vi "UHR-Fleezers Control (host) - 10.8.vi"() -> ()   [LabVIEW 2014] (continued)
            n782 = property on="Trap 1 (ON/OFF)" class="Bool (strict)"("Val(Sgnl)"=w1188) -> ()  [unwired: 2 in, 2 out]
            n783 = property on="Trap 2 (ON/OFF)" class="Bool (strict)"("Val(Sgnl)"=w1188) -> ()  [unwired: 2 in, 2 out]
            n784 = call <vilib>:"Beep.vi"() -> ()  [unwired: 3 in, 9 out]
          }
          frame #5 {
            n785 = property on="Move Cap. 2 (ADig Top)" class="Bool (strict)"("Val(Sgnl)"=TRUE ("Value (Signaling)")) -> ()  [unwired: 2 in, 2 out]
            n786 = property on="Tab Control" class="TabCtl (strict)"("Val(Sgnl)"=T4."Status" ("Value (Signaling)")) -> ()  [unwired: 2 in, 2 out]
          }
        }
      }
      event "Dip for Protein": Value Change {
        n787 = event-data() -> ()  [unwired: 1 in, 5 out]
        n788 = case shown="True" "Dip for Protein" {
          tunnel: w1194 -> [_ w1196]
          tunnel: w1193 -> [_ w1195]
          frame False {
          }
          frame True {
            n789 = while {
              tunnel: w1196 -> [w1207]
              tunnel: w1195 -> [w1206]
              i -> [w1201]
              stop <- w1203 stop-if-true
              n790 = Increment(x=w1201) -> (x+1=→"Dip #":i32)
              n791 = flat-sequence {
                tunnel: w1206 -> [w1218]
                tunnel: w1207 -> [w1219]
                tunnel: [w1219] -> w1211
                tunnel: [w1218] -> w1210
                tunnel: [w1212] -> w1197
                tunnel: [w1224] -> w1205
                tunnel: [w1225] -> w1204
                tunnel: w1211 -> [w1226]
                tunnel: w1210 -> [w1227]
                tunnel: [w1222] -> w1198
                tunnel: w1197 -> [w1222]
                tunnel: [w1235] -> w1209
                tunnel: w1205 -> [w1235]
                tunnel: [w1234] -> w1208
                tunnel: w1204 -> [w1234]
                tunnel: [w1231] -> w1202
                tunnel: [w1230] -> w1199
                tunnel: w1198 -> [w1230]
                tunnel: w1208 -> [w1255]
                tunnel: w1209 -> [w1256]
                tunnel: w1202 -> [w1257]
                tunnel: w1199 -> [w1254]
                tunnel: [w1313] -> w1203
                frame #0 {
                  n792 = local read "Trap Pos. FB ON"() -> (w1212:bool)
                  n793 = Compound Arithmetic op=AND("Flow ON\nduring dip?", "FB OFF when \nflow ON", w1212) -> (w1213:bool)
                  n794 = case shown="True" "Move trap \nbefore dip move?" {
                    frame False {
                    }
                    frame True {
                      n795 = property on="Trap Delta (MHz)" class="DigNum (strict)"("Val(Sgnl)"="Dipping Delta (MHz)") -> ()  [unwired: 2 in, 2 out]
                    }
                  }
                  n796 = property on="Green Laser ON/Interlacing" class="Bool (strict)"("Val(Sgnl)"="Green ON\nbefore dip?") -> ()  [unwired: 2 in, 2 out]
                  n797 = property on="Sample Channel\nFlow" class="Bool (strict)"("Val(Sgnl)"="Flow ON\nduring dip?") -> ()  [unwired: 2 in, 2 out]
                  n798 = case shown="True" w1213 {
                    frame False {
                    }
                    frame True {
                      n799 = property on="Trap Pos. FB ON" class="Bool (strict)"("Val(Sgnl)"=FALSE ("Value (Signaling)")) -> ()  [unwired: 2 in, 2 out]
                    }
                  }
                }
                frame #1 {
                  n800 = local read "Saved Stage Positions"() -> (w1229:dbl[][])
                  n801 = local write "Cancel dwell"(FALSE ("Cancel dwell")) -> ()
                  n802 = call "move to saved stage position.vi"("error in"=w1227, "Stage VISA resource name in"=w1226, "Position"="Dip Stage \nPosition", "Saved Stage Positions"=w1229) -> ("VISA resource name out"=w1224:refnum<visa-resource-name>, "error out"=w1225:errorcluster)
                }
                frame #2 {
                  n803 = node-c288() -> (w1233:T21)  [unwired: 4 in]
                  n804 = timed-loop {
                    timing: w1233 -> [_]
                    timing-out: [_] -> w1232
                    tunnel: [w1239] -> w1231
                    i -> [w1236]
                    stop <- w1240 stop-if-true
                    n805 = node-c288() -> ()  [unwired: 1 in, 1 out]
                    n806 = Greater Or Equal?(x=w1236, y="Dip Duration (s)") -> (x >= y?=w1248:bool)
                    n807 = local read "Dip for Protein"() -> (w1241:bool)
                    n808 = local read "Dump Beads"() -> (w1238:bool)
                    n809 = local read "Cancel dwell"() -> (w1247:bool)
                    n810 = local read "Pause dwell"() -> (w1244:bool)
                    n811 = Not(x=w1241) -> (.not. x?=w1246:bool)
                    n812 = Compound Arithmetic op=OR(w1247, w1248, w1246) -> (w1245:bool)
                    n813 = Select(t=FALSE, s=w1244, f=w1245) -> (s? t:f=w1242:bool)
                    n814 = Not(x=w1238) -> (.not. x?=w1237:bool)
                    n815 = node-c288() -> ()  [unwired: 1 in, 1 out]
                    n816 = And(x=w1241, y=w1237) -> (x .and. y?=w1239:bool)
                    n817 = Or(x=w1242, y=w1238) -> (x .or. y?=w1240:bool)
                    "Dip Time (s)" <- w1236
                  }
                  n818 = node-c288(w1232) -> ()  [unwired: 1 out]
                }
                frame #3 {
                  n819 = case shown="True" w1257 {
                    tunnel: w1256 -> [_ w1262]
                    tunnel: w1255 -> [_ w1261]
                    tunnel: w1254 -> [_ w1258]
                    frame False {
                    }
                    frame True {
                      n820 = flat-sequence {
                        tunnel: w1261 -> [w1266]
                        tunnel: w1262 -> [w1267]
                        tunnel: [w1267] -> w1260
                        tunnel: [w1266] -> w1259
                        tunnel: w1258 -> [w1263]
                        tunnel: w1260 -> [w1277]
                        tunnel: w1259 -> [w1276]
                        tunnel: w1258 -> [w1285]
                        frame #0 {
                          n821 = local read "Sample Channel\nFlow"() -> (w1265:bool)
                          n822 = case shown="False" w1265 {
                            tunnel: "Flow ON \nduring return\nfrom dip?" -> [w1268 w1271]
                            tunnel: w1263 -> [_ w1270]
                            frame False {
                              n823 = case shown="True" w1268 {
                                frame False {
                                }
                                frame True {
                                n824 = property on="Sample Channel\nFlow" class="Bool (strict)"("Val(Sgnl)"=TRUE ("Value (Signaling)")) -> ()  [unwired: 2 in, 2 out]
                                }
                              }
                            }
                            frame True {
                              n825 = case shown="False" w1271 {
                                tunnel: w1270 -> [w1272 _]
                                frame False {
                                n826 = property on="Trap Pos. FB ON" class="Bool (strict)"("Val(Sgnl)"=w1272) -> ()  [unwired: 2 in, 2 out]
                                n827 = property on="Sample Channel\nFlow" class="Bool (strict)"("Val(Sgnl)"=FALSE ("Value (Signaling)")) -> ()  [unwired: 2 in, 2 out]
                                }
                                frame True {
                                }
                              }
                            }
                          }
                        }
                        frame #1 {
                          # "For turning on green laser before stage reaches lower spot"
                          n828 = case shown="True" "Green ON\nafter start\nreturn?" {
                            frame False {
                            }
                            frame True {
                              n829 = flat-sequence {
                                frame #0 {
                                n830 = Multiply(x="Green delay after \nstart return (s)", y=1000.0) -> (x*y=w1282:dbl)
                                n831 = Wait (ms)(milliseconds to wait=w1282) -> ()  [unwired: 1 out]
                                }
                                frame #1 {
                                n832 = property on="Green Laser ON/Interlacing" class="Bool (strict)"("Val(Sgnl)"=TRUE ("Value (Signaling)")) -> ()  [unwired: 2 in, 2 out]
                                }
                              }
                            }
                          }
                          n833 = local read "Saved Stage Positions"() -> (w1280:dbl[][])
                          n834 = local write "Cancel dwell"(FALSE ("Cancel dwell")) -> ()
                          n835 = call "move to saved stage position.vi"("error in"=w1276, "Stage VISA resource name in"=w1277, "Position"="Return Stage \nPosition", "Saved Stage Positions"=w1280) -> ("error out"=w1278:errorcluster)  [unwired: 1 out]
                          n836 = local write "Stage Control Serial Error"(w1278) -> ()
                        }
                        frame #2 {
                          n837 = property on="Trap Pos. FB ON" class="Bool (strict)"("Val(Sgnl)"=w1285) -> ()  [unwired: 2 in, 2 out]
                          n838 = case shown="True" "Green ON \nafter return?" {
                            frame False {
                            }
                            frame True {
                              n839 = property on="Green Laser ON/Interlacing" class="Bool (strict)"("Val(Sgnl)"=TRUE ("Value (Signaling)")) -> ()  [unwired: 2 in, 2 out]
                            }
                          }
                          n840 = case shown="True" "Move trap after return?" {
                            frame False {
                            }
                            frame True {
                              n841 = property on="Trap Delta (MHz)" class="DigNum (strict)"("Val(Sgnl)"="Dip Trap Delta 2 (MHz)") -> ()  [unwired: 2 in, 2 out]
                            }
                          }
                          n842 = case shown="True" "Save data after return?" {
                            frame False {
                            }
                            frame True {
                              n843 = property on="Start Saving" class="Bool (strict)"("Val(Sgnl)"=TRUE ("Value (Signaling)")) -> ()  [unwired: 2 in, 2 out]
                            }
                          }
                          n844 = property on="Sample Channel\nFlow" class="Bool (strict)"("Val(Sgnl)"="Flow ON\nduring daq?") -> ()  [unwired: 2 in, 2 out]
                        }
                        frame #3 {
                          n845 = node-c288() -> (w1294:T21)  [unwired: 4 in]
                          n846 = timed-loop {
                            timing: w1294 -> [_]
                            timing-out: [_] -> w1293
                            i -> [w1295]
                            stop <- w1297 stop-if-true
                            n847 = node-c288() -> ()  [unwired: 1 in, 1 out]
                            n848 = local read "Dump Beads"() -> (w1296:bool)
                            n849 = Greater Or Equal?(x=w1295, y="Dwell Duration (s)") -> (x >= y?=w1302:bool)
                            n850 = local read "Dip for Protein"() -> (w1299:bool)
                            n851 = Not(x=w1299) -> (.not. x?=w1298:bool)
                            n852 = Compound Arithmetic op=OR(w1302, "Cancel dwell", w1298) -> (w1301:bool)
                            n853 = node-c288() -> ()  [unwired: 1 in, 1 out]
                            n854 = Select(t=FALSE, s="Pause dwell", f=w1301) -> (s? t:f=w1304:bool)
                            n855 = Or(x=w1304, y=w1296) -> (x .or. y?=w1297:bool)
                            "Dwell Time (s)" <- w1295
                          }
                          n856 = node-c288(w1293) -> ()  [unwired: 1 out]
                        }
                      }
                    }
                  }
                }
                frame #4 {
                  n857 = local read "Dip for Protein"() -> (w1314:bool)
                  n858 = local read "Dump Beads"() -> (w1311:bool)
                  n859 = local write "Cancel dwell"(FALSE ("Cancel dwell")) -> ()
                  n860 = Not(x=w1314) -> (.not. x?=w1315:bool)
                  n861 = Not(x="Cont. Repeat Dipping?") -> (.not. x?=w1317:bool)
                  n862 = Compound Arithmetic op=OR(w1315, w1317, w1311) -> (w1313:bool)
                }
              }
            }
          }
        }
      }
      event "Profile": Value Change {
        n863 = event-data() -> ()  [unwired: 1 in, 5 out]
        n864 = flat-sequence {
          tunnel: w1326 -> [w1329]
          tunnel: w1325 -> [w1337]
          tunnel: [w1331] -> w1324
          tunnel: [w1330] -> w1323
          tunnel: [w1328] -> w1321
          tunnel: [w1327] -> w1318
          tunnel: w1324 -> [w1344]
          tunnel: w1323 -> [w1343]
          tunnel: [w1341] -> w1322
          tunnel: w1321 -> [w1342]
          tunnel: [w1340] -> w1320
          tunnel: [w1339] -> w1319
          tunnel: w1318 -> [w1339]
          tunnel: w1322 -> [w1348]
          tunnel: w1320 -> [w1347]
          tunnel: w1319 -> [w1346]
          frame #0 {
            n865 = call "Read Stage Position.vi"("error in"=w1337, "VISA resource name in"=w1329) -> ("Current Position"=w1327:cluster{dbl, dbl, dbl}, "error out"=w1330:errorcluster, "VISA resource name out"=w1328:refnum<visa-resource-name>)  [unwired: 1 out]
            "Current Position" <- w1327
            n866 = local write "Stage Control Serial Error"(w1330) -> ()
            n867 = Unbundle(w1327) -> (w1334:dbl, w1336:dbl, w1332:dbl)
            n868 = Add(x=w1336, y="Y change (mm)") -> (x+y=w1333:dbl)
            n869 = Bundle(w1334, w1333, w1332) -> (w1331:cluster{dbl, dbl, dbl})  [unwired: 1 in]
          }
          frame #1 {
            # "move to new position and start saving"
            n870 = local write "Stage Moving"(TRUE ("Stage Moving")) -> ()
            n871 = local write "Start Saving"(TRUE ("Start Saving")) -> ()
            n872 = call "Set Stage Position.vi"("Position"=w1344, "error in"=w1343, "VISA resource name in"=w1342) -> ("error out"=w1340:errorcluster, "VISA resource name out"=w1341:refnum<visa-resource-name>)  [unwired: 1 out]
          }
          frame #2 {
            # "go back to start"
            n873 = call "Set Stage Position.vi"("Position"=w1346, "error in"=w1347, "VISA resource name in"=w1348) -> ()  [unwired: 3 out]
          }
          frame #3 {
            # "stop saving"
            n874 = local write "Stop Saving"(TRUE ("Stop Saving")) -> ()
            n875 = local write "Stage Moving"(FALSE ("Stage Moving")) -> ()
          }
        }
      }
      event "Move to Position 1", "Move to Position 2", "Move to Position 3", "Move to Position 4", "Move to Position 5", "Lower Ch. Cap.": Value Change {
        n876 = event-data() -> ()  [unwired: 1 in, 5 out]
        n877 = Or(x="Move to Position 5", y="Lower Ch. Cap.") -> (x .or. y?=w1354:bool)
        n878 = Build Array("Move to Position 1", "Move to Position 2", "Move to Position 3", "Move to Position 4", w1354) -> (w1357:bool[])
        n879 = Boolean Array To Number(Boolean array=w1357) -> (number=w1356:u32)
        n880 = Logarithm Base 2(1:w1356) -> (0:w1355:dbl)
        n881 = flat-sequence {
          tunnel: w1355 -> [w1366]
          tunnel: w1352 -> [w1364]
          tunnel: w1351 -> [w1363]
          frame #0 {
            n882 = local read "Saved Stage Positions"() -> (w1374:dbl[][])
            n883 = Array Subset(array=w1374, index (row)=w1366, length (row)=1 ("length"), index (col)=1 ("index"), length (col)=3 ("length")) -> (w1371:dbl[][])
            n884 = Reshape Array(w1371, 3 ("dimension size")) -> (w1369:dbl[])
            n885 = Array To Cluster(array=w1369) -> (cluster=w1368:cluster{"[0]":dbl, "[1]":dbl, "[2]":dbl})
            n886 = call "Set Stage Position.vi"("Position"=w1368, "error in"=w1363, "VISA resource name in"=w1364) -> ("error out"=w1367:errorcluster)  [unwired: 2 out]
            n887 = local write "Stage Moving"(TRUE ("Stage Moving")) -> ()
            n888 = local write "Stage Control Serial Error"(w1367) -> ()
          }
          frame #1 {
            n889 = local write "Stage Moving"(FALSE ("Stage Moving")) -> ()
            n890 = call <vilib>:"Beep.vi"() -> ()  [unwired: 3 in, 9 out]
          }
        }
      }
      event "Got ADig bead": Value Change {
        n891 = event-data() -> ()  [unwired: 1 in, 5 out]
        n892 = flat-sequence {
          frame #0 {
            n893 = local read "Cap 1 Samp Flow ON"() -> (w1378:bool)
            n894 = case shown="True" w1378 {
              frame False {
              }
              frame True {
                n895 = property on="Sample Channel\nFlow" class="Bool (strict)"("Val(Sgnl)"=TRUE ("Value (Signaling)")) -> ()  [unwired: 2 in, 2 out]
              }
            }
          }
          frame #1 {
            n896 = property on="Inject Pump 3" class="Bool (strict)"("Val(Sgnl)"=FALSE ("Value (Signaling)")) -> ()  [unwired: 2 in, 2 out]
          }
          frame #2 {
            n897 = property on="Move Cap. 1 (DNA Bottom)" class="Bool (strict)"("Val(Sgnl)"=TRUE ("Value (Signaling)")) -> ()  [unwired: 2 in, 2 out]
          }
        }
      }
      event "Force FB Data\nScript": Value Change {
        n898 = event-data() -> ()  [unwired: 1 in, 5 out]
        n899 = flat-sequence {
          tunnel: w1387 -> [w1391]
          tunnel: w1388 -> [w1392]
          tunnel: [w1392] -> w1383
          tunnel: [w1391] -> w1382
          tunnel: w1383 -> [w1395]
          tunnel: w1382 -> [w1394]
          tunnel: ["Trap Trig Fl."] -> w1384
          tunnel: [w1420] -> w1385
          tunnel: w1384 -> [w1420]
          tunnel: [w1424] -> w1386
          tunnel: w1385 -> [w1424]
          tunnel: w1386 -> [w1426]
          frame #0 {
            n900 = property on="Trap Delta (MHz)" class="DigNum (strict)"("Val(Sgnl)"="Trap Delta Before Moving") -> ()  [unwired: 2 in, 2 out]
          }
          frame #1 {
            n901 = local read "Saved Stage Positions"() -> (w1397:dbl[][])
            n902 = local write "FB Trap Pos Offset"(0.0 ("FB Trap Pos Offset")) -> ()
            n903 = property on="Trap Pos. FB Offset Factor" class="DigNum (strict)"("Val(Sgnl)"=i64 0 ("Value (Signaling)")) -> ()  [unwired: 2 in, 2 out]
            n904 = local write "Stage Moving"(TRUE ("Stage Moving")) -> ()
            n905 = call "move to saved stage position.vi"("error in"=w1394, "Stage VISA resource name in"=w1395, "Position"="Stage Position To Establish FB", "Saved Stage Positions"=w1397) -> ("error out"=w1393:errorcluster)  [unwired: 1 out]
            n906 = local write "Stage Control Serial Error"(w1393) -> ()
          }
          frame #2 {
            n907 = call <vilib>:"Beep.vi"() -> ()  [unwired: 3 in, 9 out]
            n908 = Multiply(x="Wait (s)", y=u32 1000 ("milliseconds to wait")) -> (x*y=w1403:u32)
            n909 = property on="Trap Delta (MHz)" class="DigNum (strict)"("Val(Sgnl)"="Starting \nTrap Delta (MHz)") -> ()  [unwired: 2 in, 2 out]
            n910 = local write "Stage Moving"(FALSE ("Stage Moving")) -> ()
            n911 = Wait (ms)(milliseconds to wait=w1403) -> ()  [unwired: 1 out]
            n912 = property on="Tab Control 2" class="TabCtl (strict)"("Val(Sgnl)"=T6."Feedback on Trap Position" ("Value (Signaling)")) -> ()  [unwired: 2 in, 2 out]
            n913 = property on="Tab Control" class="TabCtl (strict)"("Val(Sgnl)"=T4."Trap Control (RF)" ("Value (Signaling)")) -> ()  [unwired: 2 in, 2 out]
          }
          frame #3 {
            n914 = property on="Set Reading to\nSetpoint" class="Bool (strict)"("Val(Sgnl)"=TRUE ("Value (Signaling)")) -> ()  [unwired: 2 in, 2 out]
            n915 = Wait (ms)(milliseconds to wait=u32 500) -> ()  [unwired: 1 out]
          }
          frame #4 {
            n916 = property on="Trap Pos. FB ON" class="Bool (strict)"("Val(Sgnl)"=TRUE ("Value (Signaling)")) -> ()  [unwired: 2 in, 2 out]
            n917 = Wait (ms)(milliseconds to wait=u32 250) -> ()  [unwired: 1 out]
          }
          frame #5 {
            n918 = case shown="False" "Trap Trig Fl." {
              frame False {
                n919 = case shown="True" "Green ON after FB ON?" {
                  selector: "Green ON after FB ON?" -> [_ w1419]
                  frame False {
                  }
                  frame True {
                    n920 = property on="Green Laser ON/Interlacing" class="Bool (strict)"("Val(Sgnl)"=w1419) -> ()  [unwired: 2 in, 2 out]
                  }
                }
              }
              frame True {
              }
            }
            n921 = case shown="True" "Remove Action Offset" {
              tunnel: TRUE ("Value (Signaling)") -> [w1416 w1417]
              frame False {
                n922 = property on="Remove Unwinding Offset" class="Bool (strict)"("Val(Sgnl)"=w1416) -> ()  [unwired: 2 in, 2 out]
              }
              frame True {
                n923 = property on="Remove Action Offset" class="Bool (strict)"("Val(Sgnl)"=w1417) -> ()  [unwired: 2 in, 2 out]
              }
            }
            n924 = Wait (ms)(milliseconds to wait=u32 250) -> ()  [unwired: 1 out]
          }
          frame #6 {
            n925 = property on="Start Saving" class="Bool (strict)"("Val(Sgnl)"=TRUE ("Value (Signaling)")) -> ()  [unwired: 2 in, 2 out]
            n926 = Wait (ms)(milliseconds to wait=u32 5000) -> ()  [unwired: 1 out]
          }
          frame #7 {
            w1423 = TRUE ("Value (Signaling)")
            n927 = property on="Rem fb disp offset" class="Bool (strict)"("Val(Sgnl)"=w1423) -> ()  [unwired: 2 in, 2 out]
            n928 = property on="Remove Offset" class="Bool (strict)"("Val(Sgnl)"=w1423) -> ()  [unwired: 2 in, 2 out]
            n929 = Wait (ms)(milliseconds to wait=u32 100) -> ()  [unwired: 1 out]
          }
          frame #8 {
            n930 = case shown="True" w1426 {
              frame False {
              }
              frame True {
                n931 = local write "Trap Trig. Fl."(TRUE ("Value (Signaling)")) -> ()
              }
            }
          }
          frame #9 {
            n932 = case shown="True" "Start dipping after?" {
              frame False {
              }
              frame True {
                n933 = flat-sequence {
                  frame #0 {
                    n934 = Multiply(x="Delay before dipping (s)", y=1000.0) -> (x*y=w1430:dbl)
                    n935 = Wait (ms)(milliseconds to wait=w1430) -> ()  [unwired: 1 out]
                  }
                  frame #1 {
                    n936 = property on="Dip for Protein" class="Bool (strict)"("Val(Sgnl)"=TRUE ("Value (Signaling)")) -> ()  [unwired: 2 in, 2 out]
                    n937 = local write "Scripts"(T1."Dipping" ("Scripts")) -> ()
                  }
                }
              }
            }
          }
        }
      }
      event "Fixed Traps Data\nScript": Value Change {
        n938 = event-data() -> ()  [unwired: 1 in, 5 out]
        n939 = flat-sequence {
          frame #0 {
            n940 = case shown="True" "Green ON" {
              frame False {
              }
              frame True {
                n941 = property on="Green Laser ON/Interlacing" class="Bool (strict)"("Val(Sgnl)"=TRUE) -> ()  [unwired: 2 in, 2 out]
              }
            }
            n942 = local write "Offset (nm)"(0.0 ("Offset (nm)")) -> ()
            n943 = property on="Sample Channel\nFlow" class="Bool (strict)"("Val(Sgnl)"=FALSE ("Value (Signaling)")) -> ()  [unwired: 2 in, 2 out]
            n944 = property on="Trap Delta (MHz)" class="DigNum (strict)"("Val(Sgnl)"="Fixed Traps Trap Delta (MHz)") -> ()  [unwired: 2 in, 2 out]
          }
          frame #1 {
            n945 = Wait (ms)(milliseconds to wait=u32 1000) -> ()  [unwired: 1 out]
          }
          frame #2 {
            n946 = local write "Start Saving"(TRUE ("Start Saving")) -> ()
          }
          frame #3 {
            n947 = local read "Bead Sep. Int. Time (s)"() -> (w1441:dbl)
            n948 = Multiply(x=w1441, y=1000.0) -> (x*y=w1443:dbl)
            n949 = Wait (ms)(milliseconds to wait=w1443) -> ()  [unwired: 1 out]
          }
          frame #4 {
            n950 = property on="Remove Offset" class="Bool (strict)"("Val(Sgnl)"=TRUE ("Value (Signaling)")) -> ()  [unwired: 2 in, 2 out]
          }
          frame #5 {
            n951 = property on="Dip for Protein" class="Bool (strict)"("Val(Sgnl)"="Start dipping after?") -> ()  [unwired: 2 in, 2 out]
          }
        }
      }
      event "Got DNA bead": Value Change {
        n952 = event-data() -> ()  [unwired: 1 in, 5 out]
        n953 = flat-sequence {
          frame #0 {
            n954 = local read "Daq spot flow on"() -> (w1448:bool)
            n955 = case shown="True" w1448 {
              frame False {
              }
              frame True {
                n956 = property on="Sample Channel\nFlow" class="Bool (strict)"("Val(Sgnl)"=TRUE ("Value (Signaling)")) -> ()  [unwired: 2 in, 2 out]
              }
            }
            n957 = property on="Got DNA bead" class="Bool"("Key Focus"=FALSE) -> ()  [unwired: 2 in, 2 out]
          }
          frame #1 {
            n958 = property on="Inject Pump 1" class="Bool (strict)"("Val(Sgnl)"=FALSE ("Value (Signaling)")) -> ()  [unwired: 2 in, 2 out]
          }
          frame #2 {
            n959 = property on="Cal/Data Acq. Spot" class="Bool (strict)"("Val(Sgnl)"=TRUE ("Value (Signaling)")) -> ()  [unwired: 2 in, 2 out]
          }
        }
      }
      event "Take Stepping Data": Value Change {
        n960 = event-data() -> ()  [unwired: 1 in, 5 out]
        n961 = local read "Save ave N"() -> (w1460:dbl)
        n962 = flat-sequence {
          tunnel: w1460 -> [w1462]
          tunnel: [w1462] -> w1455
          tunnel: [w1464] -> w1456
          tunnel: w1455 -> [w1464]
          tunnel: [w1466] -> w1457
          tunnel: w1456 -> [w1466]
          tunnel: [w1469] -> w1458
          tunnel: w1457 -> [w1469]
          tunnel: [w1471] -> w1459
          tunnel: w1458 -> [w1471]
          tunnel: [w1473] -> w1453
          tunnel: w1459 -> [w1473]
          tunnel: w1453 -> [w1476]
          tunnel: [w1476] -> w1452
          tunnel: w1452 -> [w1477]
          tunnel: [w1477] -> w1454
          tunnel: w1454 -> [w1483]
          frame #0 {
            n963 = property on="Save ave N" class="DigNum (strict)"("Val(Sgnl)"="Save ave factor") -> ()  [unwired: 2 in, 2 out]
          }
          frame #1 {
            n964 = Wait (ms)(milliseconds to wait=u32 100) -> ()  [unwired: 1 out]
          }
          frame #2 {
            n965 = local read "Offset 2 Start (MHz)"() -> (w1468:dbl)
            n966 = property on="Saved AOD Raster Scan Parameter Sets" class="Arr (strict)"("Index Values"=u32[] [2]) -> ()  [unwired: 2 in, 2 out]
            n967 = property on="Trap Delta (MHz)" class="DigNum (strict)"("Val(Sgnl)"=w1468) -> ()  [unwired: 2 in, 2 out]
          }
          frame #3 {
            n968 = property on="Load parameters" class="Bool (strict)"("Val(Sgnl)"=TRUE ("Value (Signaling)")) -> ()  [unwired: 2 in, 2 out]
          }
          frame #4 {
            n969 = Wait (ms)(milliseconds to wait=u32 100) -> ()  [unwired: 1 out]
          }
          frame #5 {
            n970 = property on="Trap Raster Scan" class="Bool (strict)"("Val(Sgnl)"=TRUE ("Value (Signaling)")) -> ()  [unwired: 2 in, 2 out]
          }
          frame #6 {
            n971 = Wait (ms)(milliseconds to wait=u32 1000) -> ()  [unwired: 1 out]
          }
          frame #7 {
            n972 = while {
              stop <- w1480 stop-if-true
              n973 = local read "Raster Scanning..."() -> (w1482:bool)
              n974 = local read "Saving..."() -> (w1481:bool)
              n975 = Not(x=w1481) -> (.not. x?=w1478:bool)
              n976 = Not(x=w1482) -> (.not. x?=w1479:bool)
              n977 = And(x=w1479, y=w1478) -> (x .and. y?=w1480:bool)
            }
          }
          frame #8 {
            n978 = property on="Save ave N" class="DigNum (strict)"("Val(Sgnl)"=w1483) -> ()  [unwired: 2 in, 2 out]
          }
        }
      }
      event "Step Size (nm)": Value Change {
        n979 = event-data() -> ()  [unwired: 1 in, 5 out]
        n980 = flat-sequence {
          frame #0 {
            n981 = property on="Saved AOD Raster Scan Parameter Sets" class="Arr (strict)"("Index Values"=u32[] [1]) -> ()  [unwired: 2 in, 2 out]
          }
          frame #1 {
            n982 = Multiply(x="N Steps", y="Step Size (nm)") -> (x*y=w1485:dbl)
            n983 = property on="Scan Speed AOD (nm/s) 2" class="DigNum (strict)"("Value"="Step Size (nm)") -> ()  [unwired: 2 in, 2 out]
            n984 = property on="Step Size AOD (nm) 2" class="DigNum (strict)"("Value"="Step Size (nm)") -> ()  [unwired: 2 in, 2 out]
            n985 = property on="Scan Range AOD (nm) 2" class="DigNum (strict)"("Value"=w1485) -> ()  [unwired: 2 in, 2 out]
          }
        }
      }
      event "Take Detection Laser\nImage": Value Change {
        n986 = event-data() -> ()  [unwired: 1 in, 5 out]
        n987 = flat-sequence {
          tunnel: [w1513] -> w1503
          tunnel: [w1512] -> w1496
          tunnel: [w1511] -> w1488
          tunnel: [w1516] -> w1504
          tunnel: w1503 -> [w1516]
          tunnel: [w1515] -> w1497
          tunnel: w1496 -> [w1515]
          tunnel: [w1514] -> w1489
          tunnel: w1488 -> [w1514]
          tunnel: [w1520] -> w1505
          tunnel: w1504 -> [w1520]
          tunnel: [w1519] -> w1498
          tunnel: w1497 -> [w1519]
          tunnel: [w1518] -> w1490
          tunnel: w1489 -> [w1518]
          tunnel: [w1526] -> w1506
          tunnel: w1505 -> [w1526]
          tunnel: [w1525] -> w1499
          tunnel: w1498 -> [w1525]
          tunnel: [w1524] -> w1491
          tunnel: w1490 -> [w1524]
          tunnel: [w1530] -> w1507
          tunnel: w1506 -> [w1530]
          tunnel: [w1529] -> w1500
          tunnel: w1499 -> [w1529]
          tunnel: [w1528] -> w1492
          tunnel: w1491 -> [w1528]
          tunnel: [w1534] -> w1508
          tunnel: w1507 -> [w1534]
          tunnel: [w1533] -> w1501
          tunnel: w1500 -> [w1533]
          tunnel: [w1532] -> w1493
          tunnel: w1492 -> [w1532]
          tunnel: [w1538] -> w1509
          tunnel: w1508 -> [w1538]
          tunnel: [w1537] -> w1502
          tunnel: w1501 -> [w1537]
          tunnel: [w1536] -> w1494
          tunnel: w1493 -> [w1536]
          tunnel: w1509 -> [w1544]
          tunnel: w1502 -> [w1543]
          tunnel: [w1541] -> w1495
          tunnel: w1494 -> [w1541]
          tunnel: w1495 -> [w1545]
          frame #0 {
            n988 = local read "Green Laser ON/Interlacing"() -> (w1513:bool)
            n989 = local read "Green laser mode"() -> (w1512:enum32{"Laser ON", "Laser OFF", "Interlace"})
            n990 = local read "Green FB On/Off"() -> (w1511:bool)
          }
          frame #1 {
            n991 = property on="Green FB On/Off" class="Bool (strict)"("Val(Sgnl)"=FALSE ("Value (Signaling)")) -> ()  [unwired: 2 in, 2 out]
          }
          frame #2 {
            n992 = property on="Green Laser ON/Interlacing" class="Bool (strict)"("Val(Sgnl)"=TRUE ("Value (Signaling)")) -> ()  [unwired: 2 in, 2 out]
            n993 = property on="Flip Green Filter" class="Bool (strict)"("Val(Sgnl)"=TRUE ("Value (Signaling)")) -> ()  [unwired: 2 in, 2 out]
            n994 = property on="Green laser mode" class="RadioBtnsControl (strict)"("Val(Sgnl)"=enum32{"Laser ON", "Laser OFF", "Interlace"}."Laser ON" ("Value (Signaling)")) -> ()  [unwired: 2 in, 2 out]
          }
          frame #3 {
            n995 = Wait (ms)(milliseconds to wait=u32 500) -> ()  [unwired: 1 out]
          }
          frame #4 {
            n996 = property on="Confocal Image" class="Bool (strict)"("Val(Sgnl)"=TRUE ("Value (Signaling)")) -> ()  [unwired: 2 in, 2 out]
          }
          frame #5 {
            n997 = Wait (ms)(milliseconds to wait=u32 2000) -> ()  [unwired: 1 out]
          }
          frame #6 {
            n998 = while {
              stop <- w1539 stop-if-true
              n999 = local read "Saving..."() -> (w1540:bool)
              n1000 = Not(x=w1540) -> (.not. x?=w1539:bool)
            }
          }
          frame #7 {
            n1001 = property on="Flip Green Filter" class="Bool (strict)"("Val(Sgnl)"=TRUE ("Value (Signaling)")) -> ()  [unwired: 2 in, 2 out]
            n1002 = property on="Green Laser ON/Interlacing" class="Bool (strict)"("Val(Sgnl)"=w1544) -> ()  [unwired: 2 in, 2 out]
            n1003 = property on="Green laser mode" class="RadioBtnsControl (strict)"("Val(Sgnl)"=w1543) -> ()  [unwired: 2 in, 2 out]
          }
          frame #8 {
            n1004 = property on="Green FB On/Off" class="Bool (strict)"("Val(Sgnl)"=w1545) -> ()  [unwired: 2 in, 2 out]
          }
        }
      }
      event "Stop All": Value Change {
        n1005 = event-data() -> ()  [unwired: 1 in, 5 out]
        n1006 = local read "Stop All"() -> (w1546:bool)
      }
    }
    n1007 = node-c288() -> ()  [unwired: 1 in, 1 out]
  }
  n1008 = node-c288() -> (w94:T21)  [unwired: 4 out]
  n1009 = timed-loop "Control parameters (event loop)" {
    tunnel: w50 -> [w1555]
    shift-right: [w1554] -> _
    shift-left: errorcluster {"status"=FALSE, "code"=0, "source"=""} ("error out") -> [w1553]
    tunnel: [w1552] -> _
    timing: w92 -> [_]
    timing-out: [_] -> w91
    tunnel: w64 -> [w1551]
    tunnel: w4 -> [w1550]
    tunnel: w3 -> [w1549]
    tunnel: w2 -> [w1548]
    tunnel: w1 -> [w1547]
    stop <- w1552 stop-if-true
    n1010 = node-c288() -> ()  [unwired: 2 out]
    n1011 = event shown="[56] \"Retract Pump 3\": Value Change" {
      selector: _ -> [_ _ _ _ _ _ _ _ _ _ _ _ _ _ _ _ _ _ _ _ _ _ _ _ _ _ _ _ _ _ _ _ _ _ _ _ _ _ _ _ _ _ _ _ _ _ _ _ _ _ _ _ _ _ _ _ _ _ _ _ _ _ _ _ _ _ _ _ _ _ _ _ _]
      dyn-events: _ -> [_ _ _ _ _ _ _ _ _ _ _ _ _ _ _ _ _ _ _ _ _ _ _ _ _ _ _ _ _ _ _ _ _ _ _ _ _ _ _ _ _ _ _ _ _ _ _ _ _ _ _ _ _ _ _ _ _ _ _ _ _ _ _ _ _ _ _ _ _ _ _ _ _]
      timeout: _ -> [_ _ _ _ _ _ _ _ _ _ _ _ _ _ _ _ _ _ _ _ _ _ _ _ _ _ _ _ _ _ _ _ _ _ _ _ _ _ _ _ _ _ _ _ _ _ _ _ _ _ _ _ _ _ _ _ _ _ _ _ _ _ _ _ _ _ _ _ _ _ _ _ _]
      tunnel: w1555 -> [w1593 _ _ _ w1631 _ w1653 _ _ _ _ w1719 _ _ w1762 w1768 w1773 w1779 w1815 w1833 w1840 w1851 w1855 w1866 w1877 w1888 w1899 w1910 w1921 w1948 w2042 w2049 w2087 _ w2122 w2126 w2137 w2141 w2145 _ w2153 _ _ _ _ _ _ _ _ _ _ _ _ _ _ _ _ _ w2531 _ w2548 _ w2555 w2573 _ w2580 w2588 w2603 w2614 w2617 w2622 _ w2641]
      tunnel: [w1592 _ _ _ w1621 _ w1652 _ _ w1684 _ w1698 _ _ w1761 w1764 w1770 w1776 w1814 w1831 w1839 w1849 _ w1860 w1871 w1882 w1893 w1904 w1915 w1946 w2040 w2047 w2085 _ w2120 w2124 w2127 w2139 w2143 _ w2151 _ _ _ _ _ _ _ _ _ _ _ _ _ _ _ _ _ w2529 _ _ _ _ w2570 _ _ _ _ _ _ _ _ _] -> w1554
      tunnel: w1553 -> [w1591 _ _ _ w1630 _ w1651 _ _ w1684 _ w1718 _ _ w1760 w1763 w1769 w1775 w1813 w1832 w1838 w1850 w1854 w1865 w1876 w1887 w1898 w1909 w1920 w1947 w2041 w2048 w2086 _ w2121 w2125 w2136 w2140 w2144 _ w2152 _ _ _ _ _ _ _ _ _ _ _ _ _ _ _ _ _ w2530 _ w2547 _ w2554 w2572 _ w2579 w2587 w2602 w2613 w2616 w2621 _ w2640]
      tunnel: [_ _ _ _ _ _ _ _ _ w1683 _ _ _ _ _ _ _ _ _ _ _ _ _ _ _ _ _ _ _ _ _ _ _ _ _ _ _ _ _ _ _ _ _ _ _ _ _ _ _ _ _ _ _ _ _ _ _ _ _ _ _ _ _ _ _ _ _ _ _ _ _ _ _] -> w1552
      tunnel: [_ _ _ _ _ _ _ "Round T1 X" _ _ _ _ _ _ _ _ _ _ _ _ _ _ _ _ _ _ _ _ _ _ _ _ _ _ _ _ _ _ _ _ _ _ _ _ _ _ _ _ _ _ _ _ _ _ _ _ _ _ _ _ _ _ _ _ _ _ _ _ _ _ _ _ _] -> _
      tunnel: [_ _ _ "Adjust Scale\nto Mean" _ _ _ _ _ _ _ _ _ _ _ _ _ _ _ _ _ "Test ttrig" _ _ _ _ _ _ _ _ _ _ _ _ _ _ _ _ _ _ _ _ _ _ _ _ _ _ "Flush Sample" "Flush Pump 3" "Flush Pump 1" "Clear Volume" _ _ _ _ _ _ _ _ _ _ _ _ _ _ _ _ _ _ _ _ _] -> _
      tunnel: [_ _ _ _ _ _ _ _ "Round T2 X" _ "Delayed Interlace Start" _ _ _ _ _ _ _ _ _ _ _ _ _ _ _ _ _ _ _ _ _ _ _ _ _ _ _ _ _ _ _ _ _ _ _ _ _ _ _ _ _ _ _ _ _ _ _ _ _ _ _ _ _ _ _ _ _ _ _ _ _ _] -> _
      tunnel: w1551 -> [_ _ _ _ _ _ _ _ _ _ _ _ _ _ _ _ _ _ _ _ _ _ _ _ _ _ _ _ _ _ _ _ _ _ _ _ _ _ _ _ _ _ _ _ w2310 w2317 w2324 w2329 w2338 _ _ w2444 _ _ _ _ _ _ _ _ _ _ _ _ _ _ _ _ _ _ _ _ _]
      tunnel: w1550 -> [_ _ _ _ _ _ _ _ _ _ _ _ _ _ _ _ _ _ _ _ _ _ _ _ _ _ _ _ _ _ _ _ _ _ _ _ _ _ _ _ _ _ w2227 _ _ _ _ _ _ w2382 _ _ w2450 _ w2459 _ w2473 _ _ _ _ _ _ _ _ _ _ _ _ _ _ _ _]
      tunnel: w1549 -> [_ _ _ _ _ _ _ _ _ _ _ _ _ _ _ _ _ _ _ _ _ _ _ _ _ _ _ _ _ _ _ _ _ _ _ _ _ _ _ _ _ _ _ _ _ _ _ _ _ _ _ _ _ _ _ _ _ _ _ _ _ _ _ _ _ _ _ _ _ _ _ _ _]
      tunnel: w1548 -> [_ _ _ _ _ _ _ _ _ _ _ _ _ _ _ _ _ _ _ _ _ _ _ _ _ _ _ _ _ _ _ _ _ _ _ _ _ _ _ _ _ w2164 _ _ _ _ _ _ _ _ w2412 _ _ w2455 _ w2466 _ w2498 _ _ _ _ _ _ _ _ _ _ _ _ _ _ _]
      tunnel: w1547 -> [_ _ _ _ _ _ _ _ _ _ _ _ _ _ _ _ _ _ _ _ _ _ _ _ _ _ _ _ _ _ _ _ _ _ _ _ _ _ _ _ _ _ _ _ _ _ _ _ _ _ _ _ _ _ _ _ _ _ _ _ _ _ _ _ _ _ _ _ _ _ _ _ _]
      event "AI Count (ticks)", "Sets to FIFO (Traps)", "Save ave N", "FPGA Ave.", "# Samples/channel", "N sets to save": Value Change {
        # "So that if 'Save ave N' is updated, the AOD scanning code updates too."
        n1012 = event-data() -> ()  [unwired: 6 out]
        n1013 = local read "AI Count (ticks)"() -> (w1573:u32)
        n1014 = Boolean To (0,1)(Boolean="Sets to FIFO (Traps)") -> (0, 1=w1583:cluster{"Set 1":i16, "Set 2":i16, "Set 3":i16})
        n1015 = xnode "Read/Write Control"("FPGA VI Reference In"=w1593, "error in"=w1591, "ai count"=w1573, "AI1 Sets to FIFO"="Sets to FIFO (Traps)", "N of AI1 Int Acq Sets"="N Acq Sets (Traps + Fl.)") -> ("error out"=w1592:errorcluster)  [unwired: 1 out]
        n1016 = Cluster To Array(cluster=w1583) -> (array=w1582:i16[])
        n1017 = To Unsigned Long Integer(number=w1582) -> (unsigned 32bit integer=w1562:u32[])
        n1018 = local read "Scan steps (AOD)"() -> (w1584:u64)
        n1019 = Multiply(x=w1573, y="N Acq Sets (Traps + Fl.)") -> (x*y=w1571:u32)
        n1020 = Divide(x=40000000.0, y=w1573) -> (x/y=w1565:dbl)
        "AI rate (Hz)" <- w1565
        "Ave. Rate (Hz)" <- w1565
        n1021 = Add Array Elements(numeric array=w1562) -> (sum=w1574:u32)
        "Trap Sets" <- w1574
        n1022 = Reciprocal(x=w1565) -> (1/x=→"Ave. Period (s)":dbl)
        n1023 = property on="Scan steps (AOD)" class="DigNum (strict)"("Val(Sgnl)"=w1584) -> ()  [unwired: 2 in, 2 out]
        n1024 = Divide(x=w1565, y="N Acq Sets (Traps + Fl.)") -> (x/y=w1588:dbl)
        "Data Rate (Hz)" <- w1588
        n1025 = Reciprocal(x=w1588) -> (1/x=→"Data Period (s)":dbl)
        n1026 = local read "Save ave N"() -> (w1587:dbl)
        n1027 = Divide(x=w1588, y=w1587) -> (x/y=w1586:dbl)
        "Save Data Rate (Hz)" <- w1586
        n1028 = Reciprocal(x=w1586) -> (1/x=→"Save Data Period (s)":dbl)
        n1029 = Multiply(x=w1571, y="# Samples/trap") -> (x*y=w1569:u32)
        "Counts/DMA" <- w1569
        n1030 = property on="Trap Disp. Downsample" class="DigNum (strict)"("Maximum"="# Samples/trap") -> ()  [unwired: 2 in, 2 out]
        n1031 = Multiply(x=w1574, y="# Samples/trap") -> (x*y=w1563:u32)
        "# Samples/channel" <- w1563
        n1032 = Multiply(x=w1563, y=u32 8) -> (x*y=→"Trap AI Elements/DMA read":u32)
        n1033 = local read "APD Int. Count"() -> (w1570:u32)
        n1034 = Multiply(x=w1563, y=u32 3) -> (x*y=→"Trap Pos Elements/DMA read":u32)
        n1035 = Divide(x=w1569, y=w1570) -> (x/y=w1560:dbl)
        "APD Samples/FIFO Acq." <- w1560
        n1036 = Divide(x=w1569, y=40000000.0) -> (x/y=w1567:dbl)
        "DMA Update Period (s)" <- w1567
        n1037 = Multiply(x=2.0, y=w1560) -> (x*y=→"APD Elements/DMA read":dbl)
        n1038 = property on="APD Disp. Downsample" class="DigNum (strict)"("Maximum"=w1560) -> ()  [unwired: 2 in, 2 out]
        n1039 = local read "N sets to save"() -> (w1580:u32)
        n1040 = Multiply(x=w1567, y=w1580) -> (x*y=→"Total Time (s)":dbl)
        "FPGA Averaging" <- FALSE ("FPGA Averaging")
      }
      event "Remove Offset": Value Change {
        n1041 = event-data() -> ()  [unwired: 7 out]
        n1042 = local write "Remove Offset"(FALSE ("Remove Offset")) -> ()
        n1043 = local read "Bead Mean (nm)"() -> (w1595:dbl)
        n1044 = local read "Offset (nm)"() -> (w1596:dbl)
        n1045 = Add(x=w1595, y=w1596) -> (x+y=w1594:dbl)
        n1046 = local write "Offset (nm)"(w1594) -> ()
        n1047 = disable-structure shown="Disabled" {
          frame Disabled {
            n1048 = local read "Bead Mean (nm)"() -> (w1601:dbl)
            n1049 = Add(y=w1601) -> (x=w1600:dbl, x+y=w1599:dbl)
            n1050 = Subtract(x=w1601, y=w1600) -> (x-y=w1598:dbl)
            n1051 = property on="Bead Separation" class="WFChart (strict)"("YScale.Minimum"=w1598) -> ()  [unwired: 2 in, 2 out]
            n1052 = property on="Bead Separation" class="WFChart (strict)"("YScale.Maximum"=w1599) -> ()  [unwired: 2 in, 2 out]
          }
          frame Enabled {
          }
        }
      }
      event "Detector Type": Value Change {
        n1053 = event-data() -> ()  [unwired: 7 out]
        n1054 = local read "AI labels"() -> (w1602:string[])
        n1055 = property on="High Res. Display" class="Ring (strict)"("Strings []"=w1602) -> ()  [unwired: 2 in, 2 out]
        n1056 = Build Array (concatenate)(w1602, "none") -> (w1603:string[])
        n1057 = property on="FFT 1 Choice 1" class="Ring (strict)"("Strings []"=w1603) -> ()  [unwired: 2 in, 2 out]
        n1058 = property on="FFT 1 Choice 2" class="Ring (strict)"("Strings []"=w1603) -> ()  [unwired: 2 in, 2 out]
        n1059 = property on="FFT 2 Choice 1" class="Ring (strict)"("Strings []"=w1603) -> ()  [unwired: 2 in, 2 out]
        n1060 = property on="FFT 2 Choice 2" class="Ring (strict)"("Strings []"=w1603) -> ()  [unwired: 2 in, 2 out]
        n1061 = Bundle("APD 1", "APD 2") -> (w1606:cluster{string, string})  [unwired: 1 out]
        n1062 = Cluster To Array(cluster=w1606) -> (array=w1604:string[])
        n1063 = Build Array (concatenate)(w1604, w1603) -> (w1608:string[])
        n1064 = Array Size(array=w1608) -> (size(s)=w1609:i32)
        n1065 = property on="Signals to Plot" class="LstBox (strict)"("Item Names"=w1608) -> ()  [unwired: 2 in, 2 out]
        n1066 = property on="Signals to Plot" class="LstBox (strict)"("Number of Rows"=w1609) -> ()  [unwired: 2 in, 2 out]
        n1067 = property on="All Signals" class="WFChart (strict)"("LegNumRows"=w1609) -> ()  [unwired: 2 in, 2 out]
      }
      event "Adjust Scale\nto Mean": Value Change {
        n1068 = event-data() -> ()  [unwired: 7 out]
        n1069 = local read "APD 1 Rate (Hz)"() -> (w1618:dbl)
        n1070 = Multiply(x=1000.0, y="Above (kHz)") -> (x*y=w1616:dbl)
        n1071 = Multiply(x=1000.0, y="Below (kHz)") -> (x*y=w1614:dbl)
        n1072 = Add(x=w1616, y=w1618) -> (x+y=w1611:dbl)
        n1073 = Subtract(x=w1618, y=w1614) -> (x-y=w1612:dbl)
        n1074 = property on="APD Chart" class="WFChart (strict)"("YScale.Minimum"=w1612) -> ()  [unwired: 2 in, 2 out]
        n1075 = property on="APD Chart" class="WFChart (strict)"("YScale.Maximum"=w1611) -> ()  [unwired: 2 in, 2 out]
      }
      event "Phase adj. (AI1)", "+ phase (AI1)", "- phase (AI1)": Value Change {
        n1076 = event-data() -> ()  [unwired: 7 out]
        n1077 = Negate(x="Phase adj. (AI1)") -> (-x=w1628:i16)
        n1078 = Select(t=w1628, s="- phase (AI1)", f="Phase adj. (AI1)") -> (s? t:f=w1627:i16)
        n1079 = xnode "Read/Write Control"("FPGA VI Reference In"=w1631, "error in"=w1630, "Phase count adjustment"=w1627) -> ("FPGA VI Reference Out"=w1626:T19, "error out"=w1625:errorcluster)
        n1080 = Or(x="- phase (AI1)", y="+ phase (AI1)") -> (x .or. y?=w1622:bool)
        n1081 = xnode "Read/Write Control"("FPGA VI Reference In"=w1626, "error in"=w1625, "+ phase"=w1622) -> ("error out"=w1621:errorcluster)  [unwired: 1 out]
      }
      event "Signals to Plot": Double Click {
        w1634 = u32 9868950 ("Color Box")
        n1082 = event-data() -> ("Row"=w1636:i32)  [unwired: 9 out]
        n1083 = property on="All Signals" class="WFChart (strict)"("Active Plot"=w1636) -> (error out=w1647:errorcluster)  [unwired: 2 in, 1 out]
        n1084 = property on="All Signals" class="WFChart (strict)" props=["Plot", "Visible?", "Plot", "Plot Color"](error in=w1647) -> (error out=w1646:errorcluster, "Plot.Visible?"=w1645:bool)  [unwired: 1 in, 2 out]
        n1085 = Select(t=FALSE ("Plot.Visible"), s=w1645, f=TRUE ("Plot.Visible")) -> (s? t:f=w1640:bool)
        n1086 = property on="All Signals" class="WFChart (strict)"(error in=w1646, "Plot.Visible?"=w1640) -> (error out=w1642:errorcluster)  [unwired: 1 in, 1 out]
        n1087 = property on="All Signals" class="WFChart (strict)"(error in=w1642) -> (error out=w1637:errorcluster, "Plot.Plot Color"=w1641:u32)  [unwired: 1 in, 1 out]
        n1088 = property on="Signals to Plot" class="LstBox (strict)"(error in=w1637, "Active Row"=w1636) -> (error out=w1635:errorcluster)  [unwired: 1 in, 1 out]
        n1089 = Select(t=w1641, s=w1640, f=u32 0) -> (s? t:f=w1638:u32)
        n1090 = property on="Signals to Plot" class="LstBox (strict)"(error in=w1635, "CellFontColor"=w1638, "SelColor"=w1634, "CellBG"=w1634, "CellFontSize"=u32 20 ("Active Row:Cell Font:Size"), "CellFontBold"=TRUE ("Active Row:Cell Font:Bold")) -> ()  [unwired: 1 in, 2 out]
      }
      event "BD 1 Frequency 1 (MHz)", "BD 1 Frequency 2 (MHz)", "BD 1 Frequency 3 (MHz)", "BD 2 Frequency 1 (MHz)", "BD 2 Frequency 2 (MHz)", "BD 2 Frequency 3 (MHz)", "Trap Delta (MHz)": Value Change {
        n1091 = event-data() -> ("CtlRef"=w1650:refnum<vi>)  [unwired: 6 out]
        n1092 = control-ref of="Trap Delta (MHz)"() -> (w1649:refnum<vi>)
        n1093 = Equal?(x=w1649, y=w1650) -> (x = y?=w1648:bool)
        n1094 = case shown="False" "Oscillate Set 1" {
          tunnel: w1653 -> [w1673 _]
          tunnel: [w1672 w1676] -> w1652
          tunnel: w1651 -> [w1671 w1676]
          tunnel: w1648 -> [w1656 _]
          frame False {
            n1095 = local read "BD 1 Frequency 2 (MHz)"() -> (w1660:dbl)
            n1096 = local read "BD 1 Frequency 1 (MHz)"() -> (w1658:dbl)
            n1097 = Subtract(x=w1660, y="Trap Delta (MHz)") -> (x-y=w1657:dbl)
            n1098 = Select(t=w1657, s=w1656, f=w1658) -> (s? t:f=w1655:dbl)
            n1099 = local read "Y RF Frequency Limits (MHz)"() -> (w1661:T16)
            n1100 = local read "X RF Frequency Limits (MHz)"() -> (w1662:T16)
            n1101 = local read "BD 1 Frequency 3 (MHz)"() -> (w1674:dbl)
            n1102 = local write "BD 1 Frequency 1 (MHz)"(w1655) -> ()
            n1103 = local read "BD 2 Frequency 1 (MHz)"() -> (w1665:dbl)
            n1104 = local read "BD 2 Frequency 2 (MHz)"() -> (w1664:dbl)
            n1105 = local read "BD 2 Frequency 3 (MHz)"() -> (w1675:dbl)
            n1106 = call "set RF board frequency - interlace.vi"("Board 2 Frequency Limits"=w1661, "Board 1 Frequency Limits"=w1662, "error in"=w1671, "FPGA VI Reference In"=w1673, "Board 2 Frequency 3 (MHz)"=w1675, "Board 1 Frequency 3 (MHz)"=w1674, "Board 2 Frequency 2 (MHz)"=w1664, "Board 2 Frequency 1 (MHz)"=w1665, "Board 1 Frequency 2 (MHz)"=w1660, "Board 1 Frequency 1  (MHz)"=w1655) -> ("error out"=w1672:errorcluster)  [unwired: 1 out]
            n1107 = Subtract(x=w1665, y=w1664) -> (x-y=w1669:dbl)
            n1108 = Subtract(x=w1655, y=w1660) -> (x-y=w1670:dbl)
            n1109 = Square(x=w1669) -> (x^2=w1667:dbl)
            n1110 = Square(x=w1670) -> (x^2=w1668:dbl)
            n1111 = Add(x=w1668, y=w1667) -> (x+y=w1666:dbl)
            n1112 = Square Root(x=w1666) -> (sqrt(x)=w1663:dbl)
            n1113 = local write "Trap Delta (MHz)"(w1663) -> ()
            n1114 = property on="Initial delta (MHz)" class="DigNum (strict)"("Val(Sgnl)"=w1663) -> ()  [unwired: 2 in, 2 out]
          }
          frame True {
          }
        }
      }
      event "Round T1 X": Value Change {
        n1115 = event-data() -> ()  [unwired: 7 out]
        n1116 = local read "BD 1 Frequency 1 (MHz)"() -> (w1679:dbl)
        n1117 = Round To Nearest(number=w1679) -> (nearest integer value=w1678:dbl)
        n1118 = property on="BD 1 Frequency 1 (MHz)" class="DigNum (strict)"("Val(Sgnl)"=w1678) -> ()  [unwired: 2 in, 2 out]
      }
      event "Round T2 X": Value Change {
        n1119 = event-data() -> ()  [unwired: 7 out]
        n1120 = local read "BD 1 Frequency 2 (MHz)"() -> (w1681:dbl)
        n1121 = Round To Nearest(number=w1681) -> (nearest integer value=w1680:dbl)
        n1122 = property on="BD 1 Frequency 2 (MHz)" class="DigNum (strict)"("Val(Sgnl)"=w1680) -> ()  [unwired: 2 in, 2 out]
      }
      event "Stop All": Value Change {
        n1123 = event-data() -> ()  [unwired: 7 out]
        n1124 = local read "Stop All"() -> (w1683:bool)
      }
      event "Delayed Interlace Start": Value Change {
        n1125 = event-data() -> ()  [unwired: 7 out]
        n1126 = flat-sequence {
          frame #0 {
            n1127 = Multiply(x="Delay to Interlace (s)", y=1000.0) -> (x*y=w1686:dbl)
            n1128 = Wait (ms)(milliseconds to wait=w1686) -> ()  [unwired: 1 out]
          }
          frame #1 {
            n1129 = property on="Green laser mode" class="RadioBtnsControl (strict)"("Val(Sgnl)"=enum32{"Laser ON", "Laser OFF", "Interlace"}."Interlace" ("Value (Signaling)")) -> ()  [unwired: 2 in, 2 out]
          }
        }
      }
      event "BD 1 Amplitude 1 (%)", "BD 1 Amplitude 2 (%)", "BD 1 Amplitude 3 (%)", "BD 2 Amplitude 1 (%)", "BD 2 Amplitude 2 (%)", "BD 2 Amplitude 3 (%)", "Trap 1 ON", "Trap 2 ON", "Trap 3 ON", "Feedback On/Off", "All FB On/Off": Value Change {
        w1710 = i16 1 ("f")
        n1130 = event-data() -> ()  [unwired: 7 out]
        n1131 = local write "Trap 1 (ON/OFF)"("Trap 1 ON") -> ()
        n1132 = local write "Trap 2 (ON/OFF)"("Trap 2 ON") -> ()
        n1133 = Boolean To (0,1)(Boolean="Trap 3 ON") -> (0, 1=w1711:i16)
        n1134 = Boolean To (0,1)(Boolean="Trap 1 ON") -> (0, 1=w1712:i16)
        n1135 = Boolean To (0,1)(Boolean="Trap 2 ON") -> (0, 1=w1713:i16)
        n1136 = Select(t=w1713, s="Trap ON/OFF X or Y Amp?", f=w1710) -> (s? t:f=w1708:i16)
        n1137 = Select(t=w1712, s="Trap ON/OFF X or Y Amp?", f=w1710) -> (s? t:f=w1709:i16)
        n1138 = Select(t=w1711, s="Trap ON/OFF X or Y Amp?", f=w1710) -> (s? t:f=w1707:i16)
        n1139 = Select(t=w1710, s="Trap ON/OFF X or Y Amp?", f=w1713) -> (s? t:f=w1705:i16)
        n1140 = Select(t=w1710, s="Trap ON/OFF X or Y Amp?", f=w1712) -> (s? t:f=w1706:i16)
        n1141 = Select(t=w1710, s="Trap ON/OFF X or Y Amp?", f=w1711) -> (s? t:f=w1704:i16)
        n1142 = And(x="All FB On/Off", y="Feedback On/Off") -> (x .and. y?=w1702:cluster{"Set 1":bool, "Set 2":bool})
        n1143 = local read "BD 1 Amplitude 1 (%)"() -> (w1722:dbl)
        n1144 = local read "BD 1 Amplitude 2 (%)"() -> (w1721:dbl)
        n1145 = local read "BD 1 Amplitude 3 (%)"() -> (w1720:dbl)
        n1146 = Unbundle By Name(w1702) -> ("Set 1"=w1697:bool, "Set 2"=w1694:bool)
        n1147 = local read "Y RF Amplitude Limits (%)"() -> (w1690:T16)
        n1148 = local read "X RF Amplitude Limits (%)"() -> (w1691:T16)
        n1149 = local read "BD 2 Amplitude 1 (%)"() -> (w1723:dbl)
        n1150 = local read "BD 2 Amplitude 2 (%)"() -> (w1724:dbl)
        n1151 = local read "BD 2 Amplitude 3 (%)"() -> (w1725:dbl)
        n1152 = And(x="Trap 2 ON", y=w1694) -> (x .and. y?=w1692:bool)
        n1153 = And(x="Trap 1 ON", y=w1697) -> (x .and. y?=w1695:bool)
        n1154 = Multiply(x=w1709, y=w1722) -> (x*y=w1717:dbl)
        n1155 = Multiply(x=w1721, y=w1708) -> (x*y=w1715:dbl)
        n1156 = Multiply(x=w1720, y=w1707) -> (x*y=w1716:dbl)
        n1157 = Multiply(x=w1723, y=w1706) -> (x*y=w1726:dbl)
        n1158 = Multiply(x=w1724, y=w1705) -> (x*y=w1727:dbl)
        n1159 = Multiply(x=w1725, y=w1704) -> (x*y=w1728:dbl)
        n1160 = call "set RF board amplitude - interlace.vi"("Board 2 Amplitude Limits"=w1690, "Board 1 Amplitude Limits"=w1691, "error in"=w1718, "FPGA VI Reference In"=w1719, "Board 2 Amplitude 3 (%)"=w1728, "Board 1 Amplitude 3 (%)"=w1716, "Board 2 Amplitude 2 (%)"=w1727, "Board 2 Amplitude 1 (%)"=w1726, "Board 1 Amplitude 2 (%)"=w1715, "Board 1 Amplitude 1 (%)"=w1717) -> ("error out"=w1699:errorcluster, "FPGA VI Reference Out"=w1700:T19)
        n1161 = xnode "Read/Write Control"("FPGA VI Reference In"=w1700, "error in"=w1699, "FB On/Off Set 1"=w1695, "FB On/Off Set 2"=w1692) -> ("error out"=w1698:errorcluster)  [unwired: 1 out]
      }
      event "Load parameters": Value Change {
        n1162 = event-data() -> ()  [unwired: 7 out]
        n1163 = property on="Saved AOD Raster Scan Parameter Sets" class="Arr (strict)"() -> ("Index Values"=w1739:u32[])  [unwired: 2 in, 2 out]
        n1164 = Index Array(array=w1739, index=0) -> (element=w1736:u32)
        n1165 = local write "Load parameters"(FALSE ("Load parameters")) -> ()
        n1166 = Index Array(array="Saved AOD Raster Scan Parameter Sets", index=w1736) -> (element=w1735:T26)
        n1167 = Unbundle By Name(w1735) -> ("Scan Range AOD (nm) 2"=w1734:dbl, "Step Size AOD (nm) 2"=w1733:dbl, "Scan Speed AOD (nm/s) 2"=w1732:dbl, "Number of scans (AOD) 2"=w1731:u16)
        n1168 = flat-sequence {
          tunnel: w1734 -> [w1742]
          tunnel: w1733 -> [w1741]
          tunnel: w1732 -> [w1740]
          tunnel: w1731 -> [w1743]
          frame #0 {
            n1169 = local write "Scan Speed (nm/s)"(w1740) -> ()
            n1170 = local write "Scan Range (nm)"(w1742) -> ()
            n1171 = local write "Step Size (nm)"(w1741) -> ()
          }
          frame #1 {
            n1172 = property on="Number of F/B Scans (AOD)" class="DigNum (strict)"("Val(Sgnl)"=w1743) -> ()  [unwired: 2 in, 2 out]
          }
        }
      }
      event "Trap 1 (ON/OFF)", "Trap 2 (ON/OFF)": Value Change {
        n1173 = event-data() -> ()  [unwired: 7 out]
        n1174 = property on="Trap 2 ON" class="Bool (strict)"("Val(Sgnl)"="Trap 2 (ON/OFF)") -> ()  [unwired: 2 in, 2 out]
        n1175 = property on="Trap 1 ON" class="Bool (strict)"("Val(Sgnl)"="Trap 1 (ON/OFF)") -> ()  [unwired: 2 in, 2 out]
      }
      event "DIO count 1 (ticks)", "DIO count 2 (ticks)", "DIO count 3 (ticks)", "Interlace", "Number Interlace Sets", "Not-Interlacing Set": Value Change {
        n1176 = event-data() -> ()  [unwired: 7 out]
        n1177 = local read "DIO count 3 (ticks)"() -> (w1756:u32)
        n1178 = local read "DIO count 1 (ticks)"() -> (w1758:u32)
        n1179 = local read "DIO count 2 (ticks)"() -> (w1757:u32)
        n1180 = To Unsigned Byte Integer(number="Not-Interlacing Set") -> (unsigned 8bit integer=w1747:u8)
        n1181 = Add(x=w1747, y=u8 1) -> (x+y=w1751:u8)
        n1182 = xnode "Read/Write Control"("FPGA VI Reference In"=w1762, "error in"=w1760, "DIO count 1 (ticks)"=w1758, "DIO count 2 (ticks)"=w1757, "DIO count 3 (ticks)"=w1756, "Interlace ON/OFF"="Interlace", "Number Interlace Cycles"="Number Interlace Sets", "Interlace Off Parameters"=w1751) -> ("error out"=w1761:errorcluster)  [unwired: 1 out]
        n1183 = Build Array(w1758, w1757, w1756) -> (w1749:u32[])
        n1184 = Split 1D Array(array=w1749, index="Number Interlace Sets") -> (first subarray=w1759:u32[])  [unwired: 1 out]
        n1185 = Index Array(array=w1749, index=w1747) -> (element=w1748:u32)
        n1186 = Add Array Elements(numeric array=w1759) -> (sum=w1753:u32)
        n1187 = Select(t=w1753, s="Interlace", f=w1748) -> (s? t:f=→"Total Counts (ticks)":u32)
      }
      event "Reset Feedback": Value Change {
        n1188 = event-data() -> ()  [unwired: 7 out]
        n1189 = Unbundle By Name("Reset Feedback") -> ("Set 1"=w1766:bool, "Set 2"=w1765:bool)
        n1190 = xnode "Read/Write Control"("FPGA VI Reference In"=w1768, "error in"=w1763, "FB Reset Set 1"=w1766, "FB Reset Set 2"=w1765) -> ("error out"=w1764:errorcluster)  [unwired: 1 out]
      }
      event "PID Gains": Value Change {
        n1191 = event-data() -> ()  [unwired: 7 out]
        n1192 = Unbundle By Name("PID Gains") -> ("Set 1"=w1772:T14, "Set 2"=w1771:T14)
        n1193 = xnode "Read/Write Control"("FPGA VI Reference In"=w1773, "error in"=w1769, "FB Gains Set 1"=w1772, "FB Gains Set 2"=w1771) -> ("error out"=w1770:errorcluster)  [unwired: 1 out]
      }
      event "AI2 to Setpoint", "Setpoints (V)": Value Change {
        n1194 = event-data() -> ()  [unwired: 7 out]
        n1195 = xnode "Read/Write Control"("FPGA VI Reference In"=w1779, "error in"=w1775) -> ("FPGA VI Reference Out"=w1778:T19, "error out"=w1777:errorcluster, "AI2 Y Sum Set 1"=w1786, "AI2 Y Sum Set 2"=w1785)
        n1196 = Cluster To Array(cluster="AI2 to Setpoint") -> (array=w1789:bool[])
        n1197 = local read "AI2 (V)"() -> (w1787:cluster{"Set 1":dbl, "Set 2":dbl})
        n1198 = Or Array Elements(Boolean array=w1789) -> (logical OR=w1790:bool)
        n1199 = Bundle By Name(cluster=w1787, "Set 1"=w1786, "Set 2"=w1785) -> (w1784:cluster{"Set 1":dbl, "Set 2":dbl})
        n1200 = Divide(x=w1784, y=3276.7) -> (x/y=w1783:cluster{"Set 1":dbl, "Set 2":dbl})
        "AI2 (V)" <- w1783
        n1201 = case shown="True" w1790 {
          tunnel: [w1793 w1810] -> w1782
          tunnel: "AI2 to Setpoint" -> [_ w1806]
          tunnel: "Setpoints (V)" -> [w1794 w1809]
          tunnel: w1783 -> [_ w1803]
          frame False {
            n1202 = Multiply(x=3276.7, y=w1794) -> (x*y=w1795:cluster{"Set 1":dbl, "Set 2":dbl})
            n1203 = To Word Integer(number=w1795) -> (16bit integer=w1793:cluster{"Set 1":i16, "Set 2":i16})
          }
          frame True {
            n1204 = Unbundle By Name(w1803) -> ("Set 1"=w1802:dbl, "Set 2"=w1801:dbl)
            n1205 = Unbundle By Name(w1809) -> ("Set 1"=w1808:dbl, "Set 2"=w1807:dbl)
            n1206 = Unbundle By Name(w1806) -> ("Set 1"=w1805:bool, "Set 2"=w1804:bool)
            n1207 = Select(t=w1802, s=w1805, f=w1808) -> (s? t:f=w1800:dbl)
            n1208 = Select(t=w1801, s=w1804, f=w1807) -> (s? t:f=w1799:dbl)
            n1209 = Bundle By Name(cluster=w1809, "Set 1"=w1800, "Set 2"=w1799) -> (w1797:cluster{"Set 1":dbl, "Set 2":dbl})
            n1210 = local write "Setpoints (V)"(w1797) -> ()
            n1211 = Multiply(x=3276.7, y=w1797) -> (x*y=w1798:cluster{"Set 1":dbl, "Set 2":dbl})
            n1212 = To Word Integer(number=w1798) -> (16bit integer=w1810:cluster{"Set 1":i16, "Set 2":i16})
          }
        }
